vi "Pressure_control_subVI _V2.vi"(7 "Run Sequence":bool, 8 "user sequence, present (s) in, current step in, seq time in":T6, 9 "pressure parameters in":T1={"valve % open"=100.0, "Desired pressure"=0.0, "set Vapor sccm"=0.0, "set Gas sccm"=0.0, "Valve mode"=enum."% Open", "Pressure Mode"=enum."Abs. pressure", "analyte partial pressure"=100.0, "Turbo pump\nauto on"=TRUE} caption="Set pressure parameters" {"analyte partial pressure" min=0.0 max=100.0 step=5.0; "set Gas sccm" min=0 max=200 step=5; "set Vapor sccm" min=0 max=200 step=5; "Desired pressure" min=0.0 max=760.0 step=5.0; "valve % open" min=0.0 max=100.0 step=5.0 format="%#_2f"}, 10 "Jump to next step":bool, 11 "pressure control on? / DAQ IDs/errors in":T5) -> (0 "current step # out, shift register time out, seq button on?":T3, 1 "sequence over? USE THIS TO REINITIALIZE RUN SEQUENCE BUTTON SO PROGRAM ENDS":bool, 2 "save press/RH/gasflow/vaporflow - read valve position/pressure/vaporflow/gasflow":T2, 3 "pressure control on out, DAQ IDs/errors out":T4, 4 "sequence end date/time string":string, 5 "pressure_setpoint":string)   [LabVIEW 2014]
uses:
  <vilib>/DAQmx/read.llb/DAQmx Read (Analog 1D DBL NChan 1Samp).vi
  <vilib>/DAQmx/write.llb/DAQmx Write (Analog 1D DBL NChan 1Samp).vi
  <vilib>/DAQmx/write.llb/DAQmx Write (Digital Bool 1Line 1Point).vi
panel:
  # "100%"
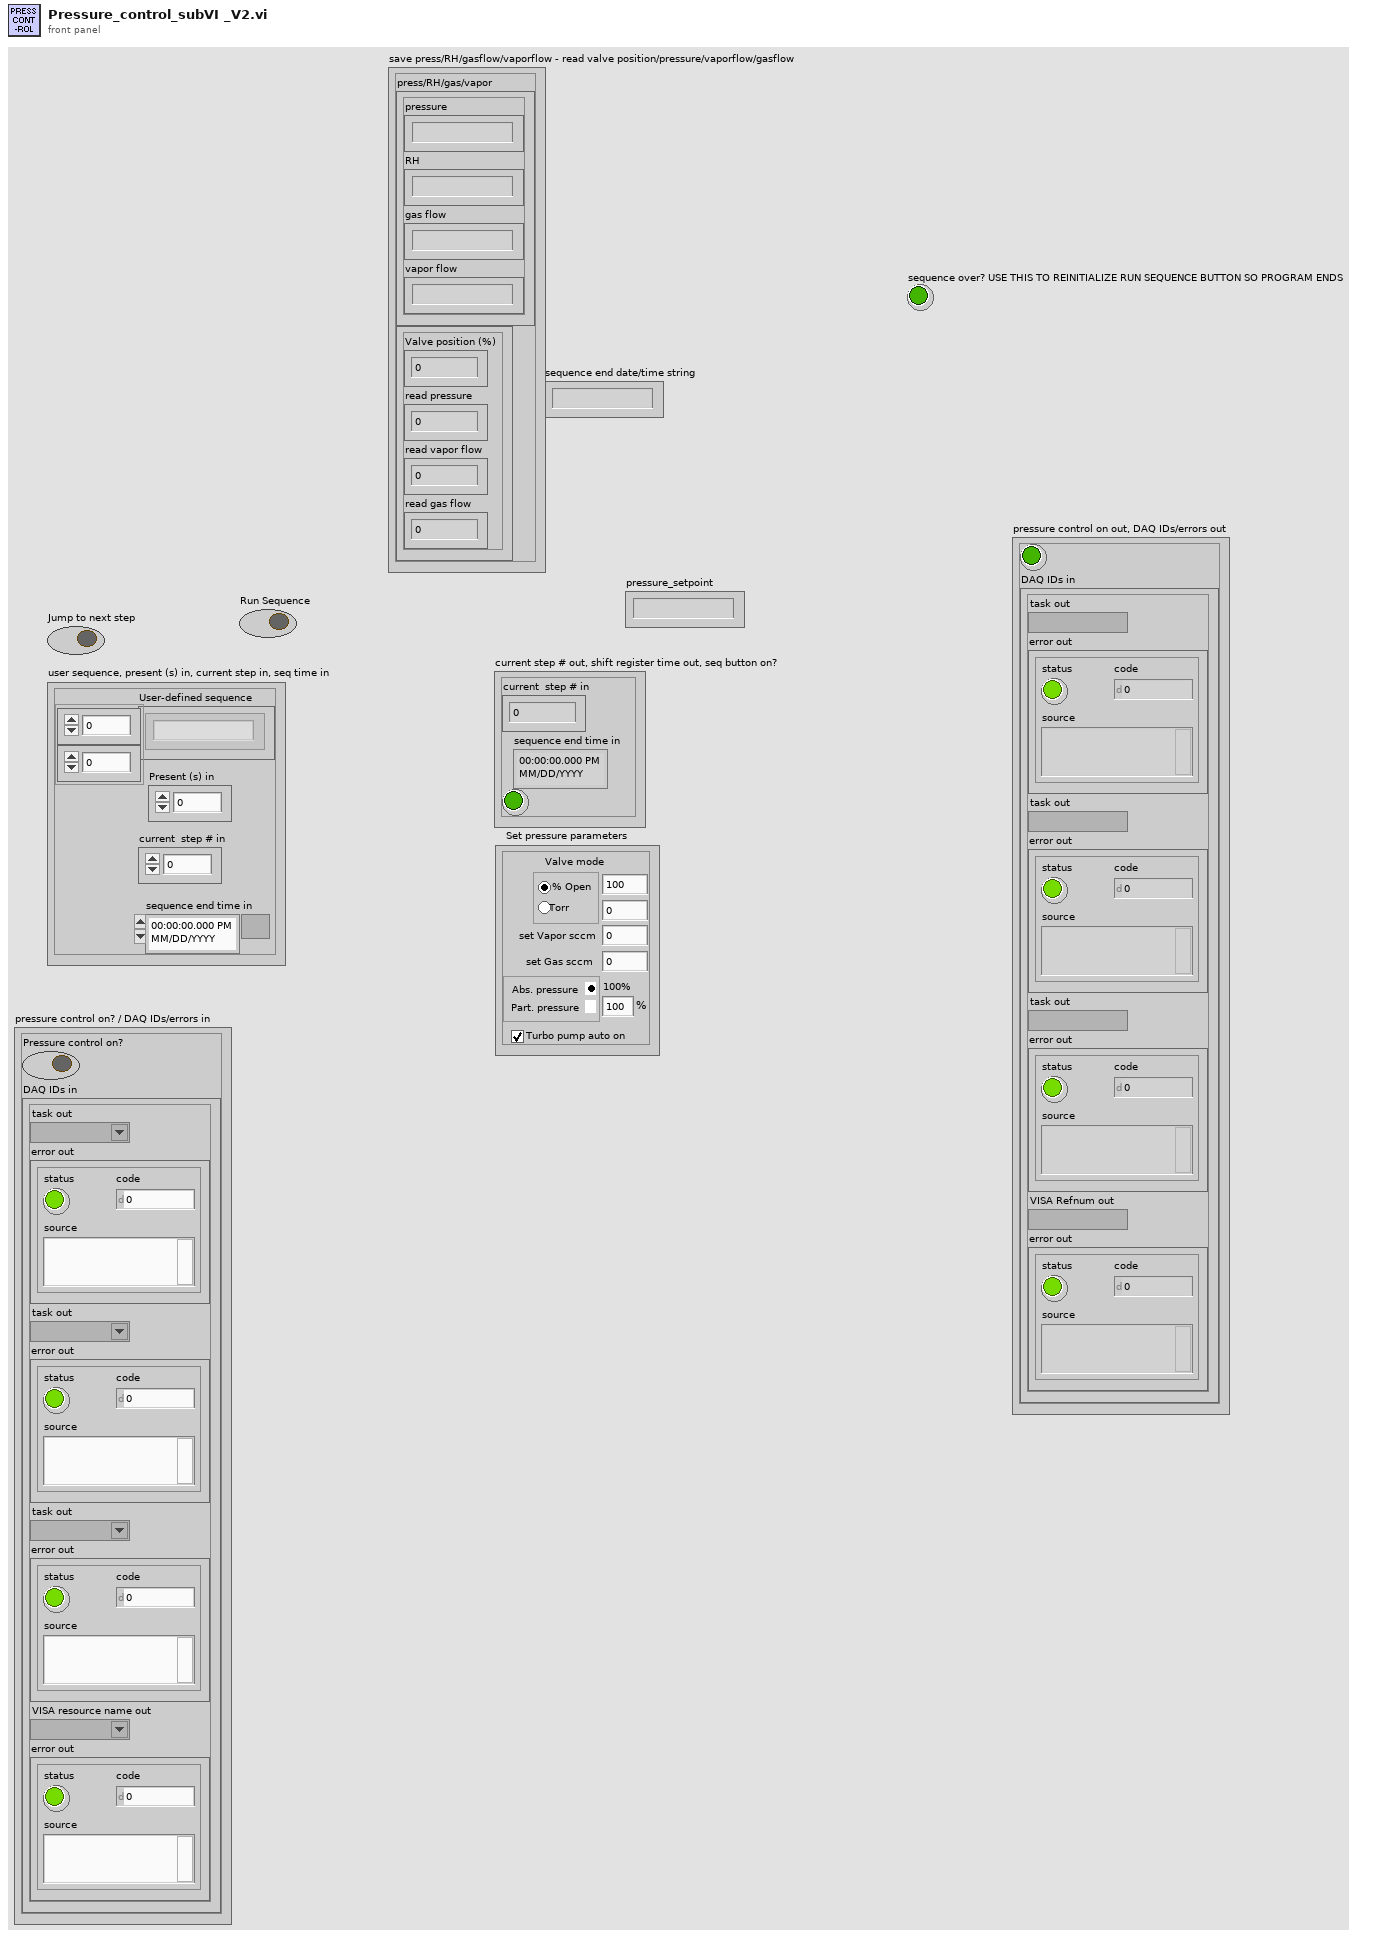
[diagram p1: front panel]
types:
  T1 = cluster{"valve % open":dbl, "Desired pressure":dbl, "set Vapor sccm":sgl, "set Gas sccm":sgl, "Valve mode":enum32{"% Open", "Torr "}, "Pressure Mode":enum32{"Abs. pressure", " Part. pressure"}, "analyte partial pressure":dbl, "Turbo pump\nauto on":bool}
  T2 = cluster{"press/RH/gas/vapor":cluster{"pressure":string, "RH":string, "gas flow":string, "vapor flow":string}, "Cluster":cluster{"Valve position (%)":dbl, "read pressure":dbl, "read vapor flow":dbl, "read gas flow":dbl}}
  T3 = cluster{"current  step # in":i32, "sequence end time in":timestamp, "Boolean":bool}
  T4 = cluster{"Boolean":bool, "DAQ IDs in":cluster{"task out":refnum<k21>, "error out":errorcluster, "task out":refnum<k21>, "error out":errorcluster, "task out":refnum<k21>, "error out":errorcluster, "VISA Refnum out":refnum<visa-resource-name>, "error out":errorcluster}}
  T5 = cluster{"Pressure control on?":bool, "DAQ IDs in":cluster{"task out":refnum<k21>, "error out":errorcluster, "task out":refnum<k21>, "error out":errorcluster, "task out":refnum<k21>, "error out":errorcluster, "VISA resource name out":refnum<visa-resource-name>, "error out":errorcluster}}
  T6 = cluster{"User-defined sequence":string[][], "Present (s) in":dbl, "current  step # in":i32, "sequence end time in":timestamp}
  T7 = cluster{"task out":refnum<k21>, "error out":errorcluster, "task out":refnum<k21>, "error out":errorcluster, "task out":refnum<k21>, "error out":errorcluster, "VISA resource name out":refnum<visa-resource-name>, "error out":errorcluster}
  T8 = cluster{"Valve position (%)":dbl, "pressure":dbl, "vapor flow":dbl, "gas flow":dbl}
  T9 = cluster{"pressure":string, "RH":string, "gas flow":string, "vapor flow":string}
  T10 = cluster{"String":dbl, "String":dbl, "Pressure Control":u32}
  T11 = cluster{"Valve position (%)":dbl, "read pressure":dbl, "read vapor flow":dbl, "read gas flow":dbl}
  T12 = cluster{"task out":refnum<k21>, "error out":errorcluster, "task out":refnum<k21>, "error out":errorcluster, "task out":refnum<k21>, "error out":errorcluster, "VISA Refnum out":refnum<visa-resource-name>, "error out":errorcluster}
  T13 = cluster{"press/RH/gas/vapor":cluster{"pressure":string, "RH":string, "gas flow":string, "vapor flow":string}, cluster{"Valve position (%)":dbl, "read pressure":dbl, "read vapor flow":dbl, "read gas flow":dbl}}
  T14 = cluster{"current  step # in":i32, "sequence end time in":timestamp, bool}
  T15 = cluster{bool, "DAQ IDs in":cluster{"task out":refnum<k21>, "error out":errorcluster, "task out":refnum<k21>, "error out":errorcluster, "task out":refnum<k21>, "error out":errorcluster, "VISA Refnum out":refnum<visa-resource-name>, "error out":errorcluster}}
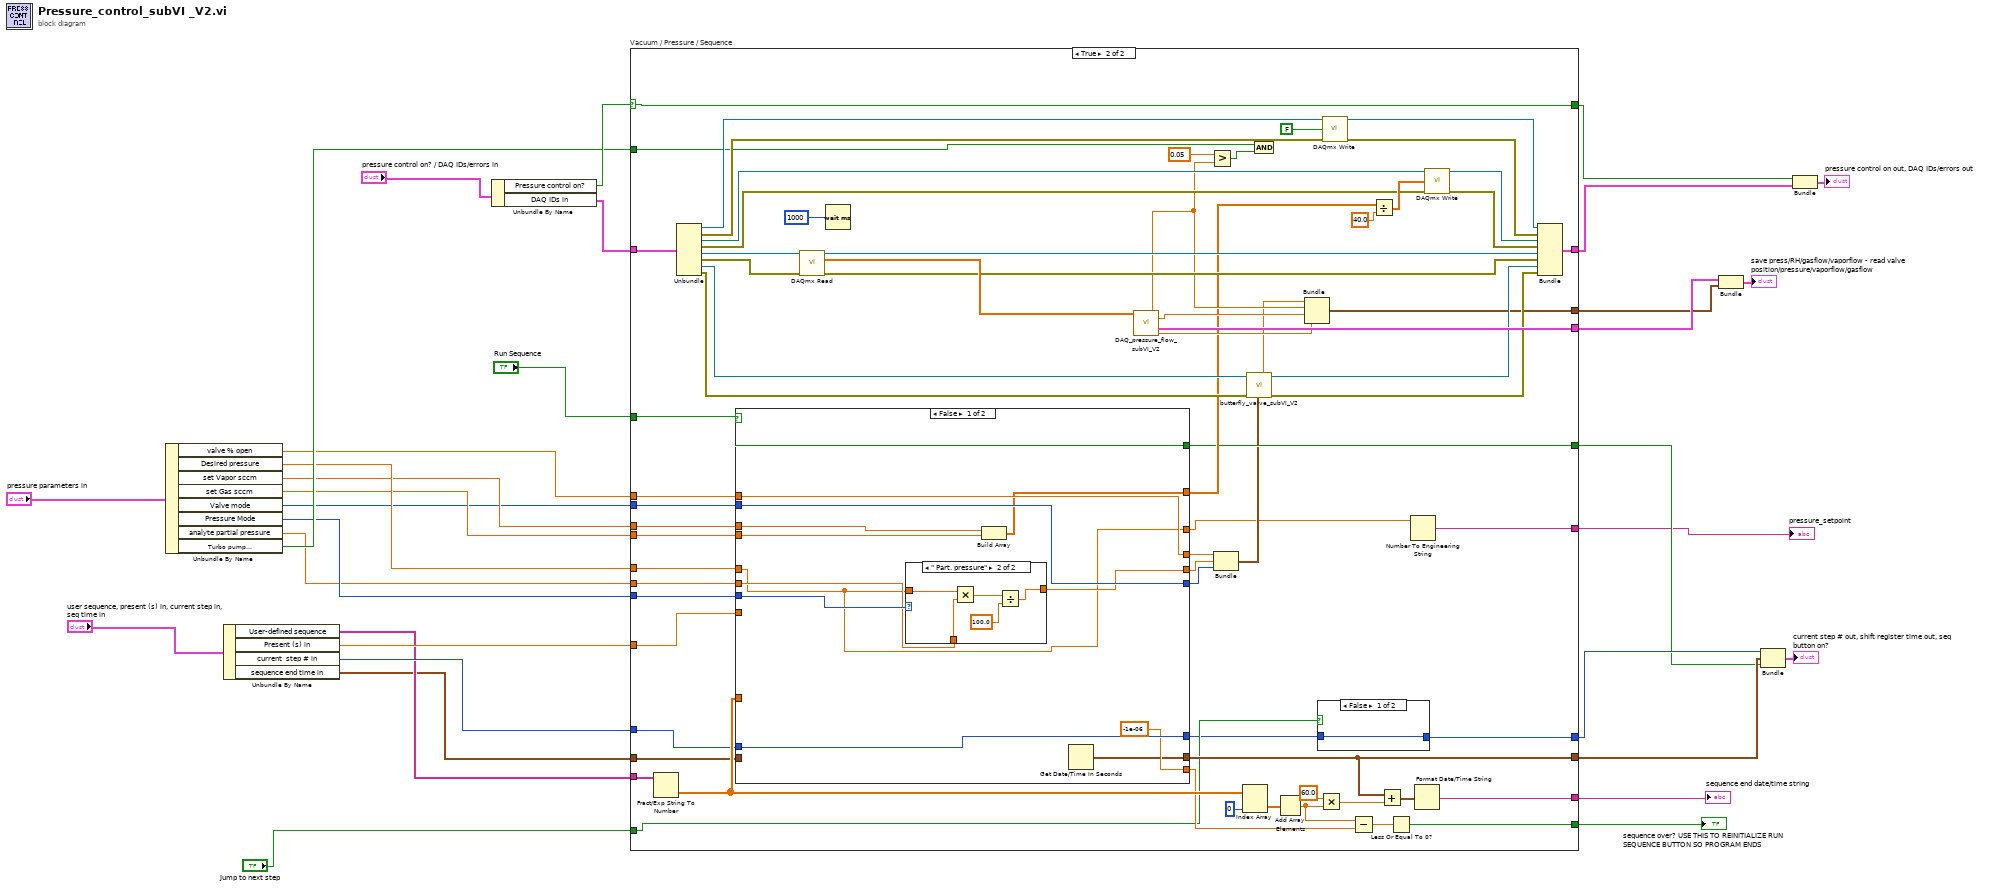
[diagram p0: block diagram]
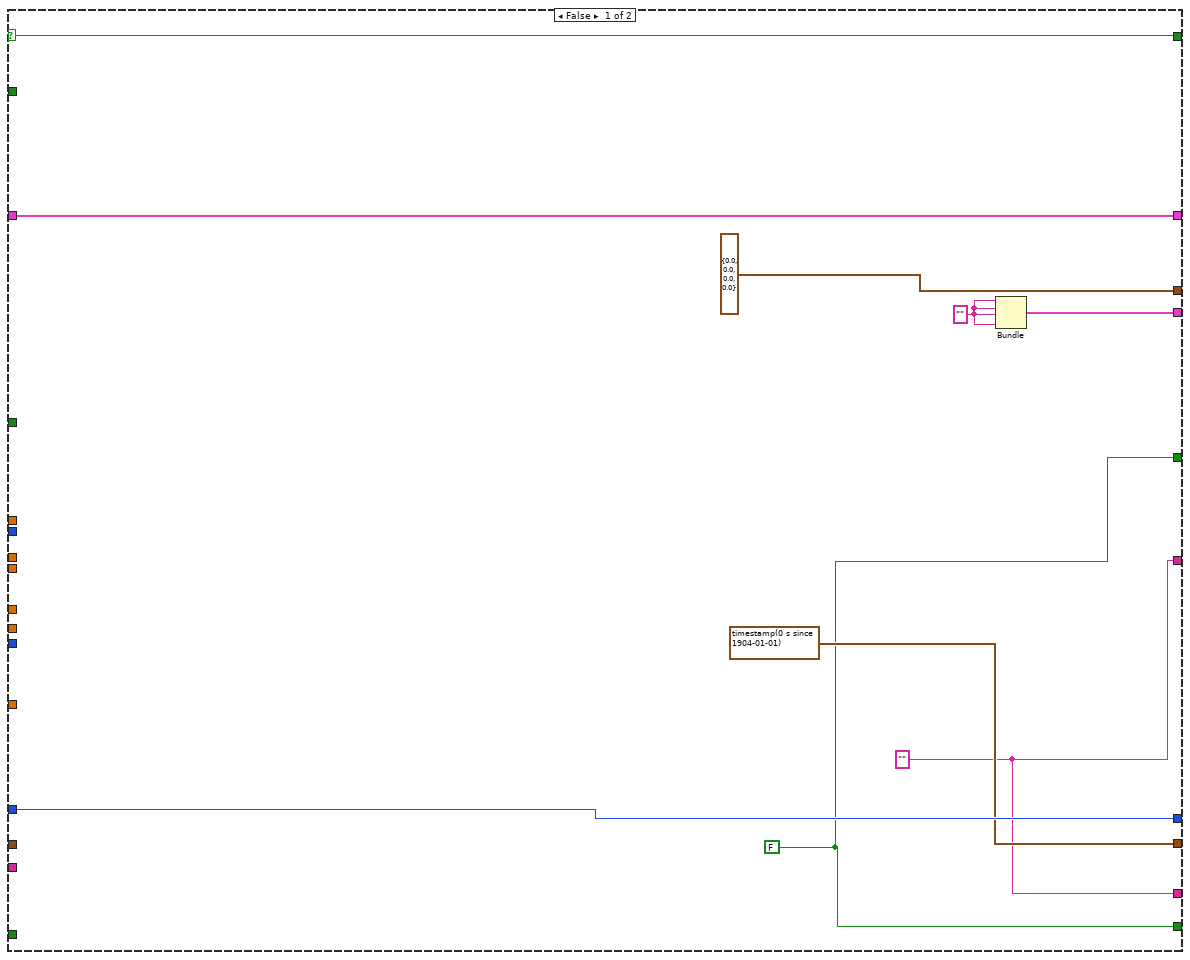
[diagram p2: hidden frame]
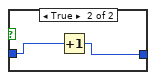
[diagram p3: hidden frame]
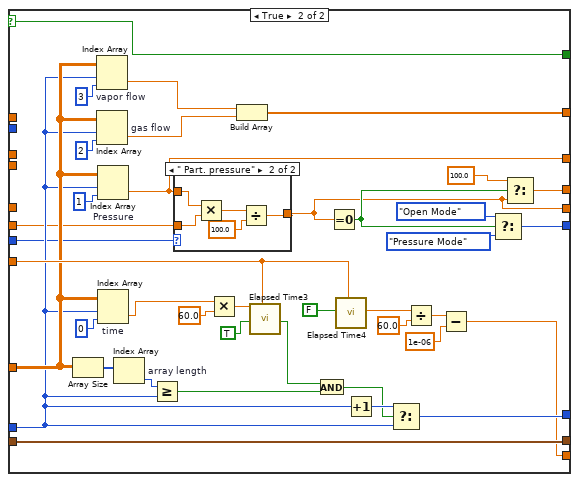
[diagram p5: hidden frame]
diagram:
  n1 = Unbundle By Name("pressure parameters in") -> ("valve % open"=w3:dbl, "Desired pressure"=w7:dbl, "set Vapor sccm"=w5:sgl, "set Gas sccm"=w6:sgl, "Valve mode"=w4:enum32{"% Open", "Torr "}, "Pressure Mode"=w9:enum32{"Abs. pressure", " Part. pressure"}, "analyte partial pressure"=w8:dbl, "Turbo pump\nauto on"=w10:bool)
  n2 = Unbundle By Name("user sequence, present (s) in, current step in, seq time in") -> ("User-defined sequence"=w26:string[][], "Present (s) in"=w27:dbl, "current  step # in"=w28:i32, "sequence end time in"=w25:timestamp)
  n3 = Unbundle By Name("pressure control on? / DAQ IDs/errors in") -> ("Pressure control on?"=w22:bool, "DAQ IDs in"=w23:T7)
  n4 = case "Vacuum / Pressure / Sequence" shown="True" w22 {
    selector: w22 -> [w34 w52]
    tunnel: w23 -> [w37 w105]
    tunnel: w28 -> [w41 w68]
    tunnel: [w41 w45] -> w18
    tunnel: [w35 w66] -> w16
    tunnel: [timestamp(0 s since 1904-01-01) ("seconds since 1Jan1904") w65] -> w17
    tunnel: [w39 w86] -> w14
    tunnel: [w37 w77] -> w20
    tunnel: w10 -> [_ w74]
    tunnel: w26 -> [_ w73]
    tunnel: [w33 w72] -> w32
    tunnel: [T8 {"Valve position (%)"=0.0, "pressure"=0.0, "vapor flow"=0.0, "gas flow"=0.0} w71] -> w13
    tunnel: w27 -> [_ w63]
    tunnel: "Run Sequence" -> [_ w62]
    tunnel: w25 -> [_ w61]
    tunnel: [w35 w60] -> w30
    tunnel: w7 -> [_ w59]
    tunnel: w3 -> [_ w58]
    tunnel: w5 -> [_ w57]
    tunnel: w9 -> [_ w56]
    tunnel: w4 -> [_ w55]
    tunnel: w6 -> [_ w54]
    tunnel: w8 -> [_ w53]
    tunnel: [w34 w52] -> w21
    tunnel: "Jump to next step" -> [_ w47]
    tunnel: [w33 w42] -> w1
    frame False {
      w33 = "" ("date/time string")
      w35 = FALSE
      w38 = ""
      n5 = Bundle(w38, w38, w38, w38) -> (w39:cluster{string, string, string, string})  [unwired: 1 in]
    }
    frame True {
      n6 = Fract/Exp String To Number ("user sequence")(string=w73) -> (number=w69:dbl[][])  [unwired: 3 in, 1 out]
      n7 = Unbundle(w105) -> ("task out"=w98:refnum<k21>, "error out"=w97:errorcluster, "task out"=w99:refnum<k21>, "error out"=w100:errorcluster, "task out"=w101:refnum<k21>, "error out"=w102:errorcluster, "VISA resource name out"=w103:refnum<visa-resource-name>, "error out"=w104:errorcluster)
      n8 = case "Sequence" shown="False" w62 {
        selector: w62 -> [w122 w151]
        tunnel: w63 -> [_ w159]
        tunnel: [w125 w160] -> w46
        tunnel: w68 -> [w125 w152]
        tunnel: w54 -> [w120 _]
        tunnel: [w117 w132] -> w51
        tunnel: w69 -> [_ w154]
        tunnel: w55 -> [w124 _]
        tunnel: [w124 w137] -> w50
        tunnel: [-1e-06 w134] -> w64
        tunnel: [w122 w151] -> w66
        tunnel: [w121 w141] -> w44
        tunnel: w58 -> [w121 _]
        tunnel: [w119 w147] -> w67
        tunnel: [w118 w146] -> w65
        tunnel: w61 -> [_ w146]
        tunnel: w59 -> [w113 _]
        tunnel: w53 -> [w114 w145]
        tunnel: w56 -> [w116 w143]
        tunnel: w57 -> [w115 _]
        tunnel: [w113 w133] -> w43
        frame False {
          n9 = case shown="\" Part. pressure\"" w116 {
            tunnel: [w126 w127] -> w117
            tunnel: w113 -> [w126 w129]
            tunnel: w114 -> [_ w128]
            frame "Abs. pressure", Default {
            }
            frame " Part. pressure" {
              n10 = Multiply(x=w129, y=w128) -> (x*y=w131:dbl)
              n11 = Divide(x=w131, y=100.0 ("Analyte part. press. (%)")) -> (x/y=w127:dbl)
            }
          }
          n12 = Build Array(w115, w120) -> (w119:sgl[])
          n13 = Get Date/Time In Seconds() -> (seconds since 1Jan1904=w118:timestamp)
        }
        frame True {
          n14 = Array Size(array=w154) -> (size(s)=w170:i32[])
          n15 = Index Array "vapor flow"(array=w154, index (row)=w152, index (col)=3 ("disabled index (col)")) -> (element=w149:dbl)
          n16 = Index Array "gas flow"(array=w154, index (row)=w152, index (col)=2 ("disabled index (col)")) -> (element=w148:dbl)
          n17 = Index Array "Pressure"(array=w154, index (row)=w152, index (col)=1 ("disabled index (col)")) -> (element=w133:dbl)
          n18 = Index Array "time"(array=w154, index (row)=w152, index (col)=0) -> (element=w163:dbl)
          n19 = Index Array "array length"(array=w170) -> (element=w155:i32)  [unwired: 1 in]
          n20 = Greater Or Equal?(x=w155, y=w152) -> (x >= y?=w167:bool)
          n21 = case shown="\" Part. pressure\"" w143 {
            tunnel: [w171 w172] -> w132
            tunnel: w133 -> [w171 w174]
            tunnel: w145 -> [_ w173]
            frame "Abs. pressure", Default {
            }
            frame " Part. pressure" {
              n22 = Multiply(x=w174, y=w173) -> (x*y=w175:dbl)
              n23 = Divide(x=w175, y=100.0 ("Analyte part. press. (%)")) -> (x/y=w172:dbl)
            }
          }
          n24 = Multiply(x=w163, y=60.0) -> (x*y=w153:dbl)
          n25 = Build Array(w149, w148) -> (w147:dbl[])
          n26 = call "Elapsed Time3"("Time Target (s)"=w153, "Auto Reset"=TRUE, "Set Start Time (s)"=w159) -> ("Time has Elapsed"=w144:bool)  [unwired: 9 in, 7 out]
          n27 = And(x=w144, y=w167) -> (x .and. y?=w150:bool)
          n28 = Equal To 0?(x=w132) -> (x = 0?=w140:bool)
          n29 = call "Elapsed Time4"("Reset"=FALSE, "Set Start Time (s)"=w159) -> ("Elapsed Time (s)"=w157:dbl)  [unwired: 10 in, 7 out]
          n30 = Increment(x=w152) -> (x+1=w161:i32)
          n31 = Select(t=w161, s=w150, f=w152) -> (s? t:f=w160:i32)
          n32 = Divide(x=w157, y=60.0) -> (x/y=w136:dbl)
          n33 = Subtract(x=w136, y=1e-06) -> (x-y=w134:dbl)
          n34 = Select(t=enum32{"Open Mode", "Pressure Mode"}."Open Mode" ("Pressure Control"), s=w140, f=enum32{"Open Mode", "Pressure Mode"}."Pressure Mode" ("Pressure Control")) -> (s? t:f=w137:enum32{"Open Mode", "Pressure Mode"})
          n35 = Select(t=100.0 ("valve % open 2"), s=w140, f=w132) -> (s? t:f=w141:dbl)
        }
      }
      n36 = call-poly <vilib>:"DAQmx Read.vi"("task/channels in"=w101, "error in"=w102) -> ("task out"=w81:refnum<k21>, "data"=w108:dbl[], "error out"=w80:errorcluster)  [unwired: 11 in]
      n37 = Wait (ms)(milliseconds to wait=u32 1000) -> ()  [unwired: 1 out]
      n38 = call "DAQ_pressure_flow_subVI_V2.vi"("vac press"=w108) -> ("read pressure"=w70:dbl, "read vapor flow"=w76:dbl, "press/RH/gas/vapor"=w86:T9, "read gas flow"=w75:dbl)  [unwired: 11 in]
      n39 = Greater?(x=0.05, y=w70) -> (0:w87:bool)
      n40 = Bundle("String"=w44, "String"=w51, "Pressure Control"=w50) -> (w48:T10)  [unwired: 1 in]
      n41 = Index Array(array=w69, index (col)=0 ("disabled index (col)")) -> (element=w95:dbl[])  [unwired: 1 in]
      n42 = call "butterfly_valve_subVI_V2.vi"("% open / desired pressure / pressure mode"=w48, "error in (no error)"=w104, "VISA Refnum in"=w103) -> ("error out"=w78:errorcluster, "VISA Refnum out"=w79:refnum<visa-resource-name>, "Valve position (%)"=w49:dbl)  [unwired: 6 in]
      n43 = And(x=w74, y=w87) -> ()  [unwired: 1 out]
      n44 = Add Array Elements(numeric array=w95) -> (sum=w89:dbl)
      n45 = Bundle("Valve position (%)"=w49, "read pressure"=w70, "read vapor flow"=w76, "read gas flow"=w75) -> (w71:T11)  [unwired: 1 in]
      n46 = case shown="False" w47 {
        tunnel: w46 -> [w110 w112]
        tunnel: [w110 w111] -> w45
        frame False {
        }
        frame True {
          n47 = Increment(x=w112) -> (x+1=w111:i32)
        }
      }
      n48 = Multiply(x=60.0 ("y"), y=w89) -> (x*y=w91:dbl)
      n49 = call-poly <vilib>:"DAQmx Write.vi"("task/channels in"=w98, "data"=FALSE, "error in"=w97) -> ("task out"=w85:refnum<k21>, "error out"=w84:errorcluster)  [unwired: 10 in, 1 out]
      n50 = Subtract(x=w89, y=w64) -> (x-y=w93:dbl)
      n51 = Divide(x=w67, y=40.0 ("Waveform")) -> (x/y=w107:dbl[])
      n52 = Add(x=w65, y=w91) -> (x+y=w90:timestamp)
      n53 = Less Or Equal To 0?(x=w93) -> (x <= 0?=w60:bool)
      n54 = Number To Engineering String(4:w43) -> (0:w42:string)  [unwired: 3 in]
      n55 = Format Date/Time String(seconds (now)=w90) -> (date/time string=w72:string)  [unwired: 2 in]
      n56 = call-poly <vilib>:"DAQmx Write.vi"("task/channels in"=w99, "data"=w107, "error in"=w100) -> ("task out"=w83:refnum<k21>, "error out"=w82:errorcluster)  [unwired: 10 in, 1 out]
      n57 = Bundle("task out"=w85, "error out"=w84, "task out"=w83, "error out"=w82, "task out"=w81, "error out"=w80, "VISA Refnum out"=w79, "error out"=w78) -> (w77:T12)  [unwired: 1 in]
    }
  }
  "sequence end date/time string" <- w32
  "sequence over? USE THIS TO REINITIALIZE RUN SEQUENCE BUTTON SO PROGRAM ENDS" <- w30
  "pressure_setpoint" <- w1
  n58 = Bundle("press/RH/gas/vapor"=w14, w13) -> (→"save press/RH/gasflow/vaporflow - read valve position/pressure/vaporflow/gasflow":T13)  [unwired: 1 in]
  n59 = Bundle("current  step # in"=w18, "sequence end time in"=w17, w16) -> (→"current step # out, shift register time out, seq button on?":T14)  [unwired: 1 in]
  n60 = Bundle(w21, "DAQ IDs in"=w20) -> (→"pressure control on out, DAQ IDs/errors out":T15)  [unwired: 1 in]
